vi "G# - SupportMethods.vi"() -> ()   [LabVIEW 2017]
doc: "Support Methods\nThis example demonstrates the use of the G#Object support methods that is always applicable for all G# objects.\n\nBy using the G# Debugger found in Tools->G# Debugger a text log can be followed showing how the objects were created and destroyed."
uses:
  MyDemoClass_class/MyDemoClass.lvclass
  C:/Program Files/National Instruments/LabVIEW 2017/vi.lib/addons/_AddQ/G#Object/G#Object.lvclass
  vi.lib/addons/_AddQ/G#Object/G#Object.lvclass
panel:
  in  "error in (no error)":errorcluster
  out "nr of objects":i32
  out "object name":string
  out "is empty?":bool
  out "string 2":string
  out "string 1":string
  out "is equal 1":bool
  out "is equal 2":bool
  out "class name 2":string
  out "class name 1":string
  out "object ID 2":u32 format="%x"
  out "object ID 1":u32 format="%x"
  out "is instance of":bool
  out "not a refnum? 1":bool
  out "not a refnum? 2":bool
  out "not a refnum? 3":bool
  out "class name 3":string
  out "class path":path
  out "error out":errorcluster
  # "Support Methods\nThis example demonstrates the use of the G#Object support methods that is always applicable for all G# objects.\n\nBy using the G# Debugger found in Tools->G# Debugger a text log can be followed showing how the objects were created and destroyed."
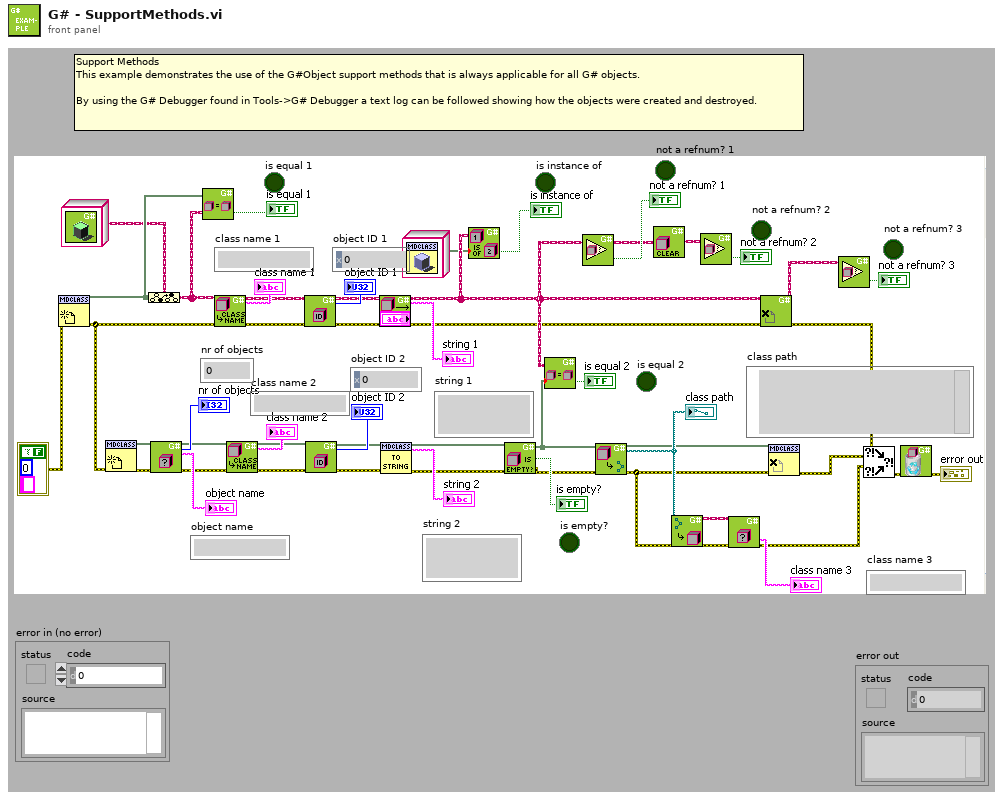
[diagram p1: front panel]
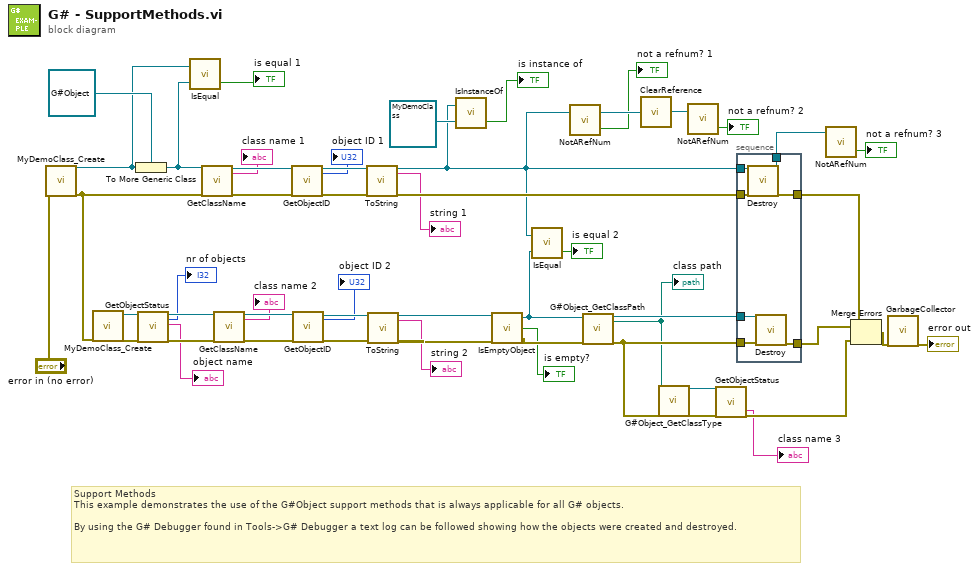
[diagram p0: block diagram]
diagram:
  # "Support Methods\nThis example demonstrates the use of the G#Object support methods that is always applicable for all G# objects.\n\nBy using the G# Debugger found in Tools->G# Debugger a text log can be followed showing how the objects were created and destroyed."
  n1 = call "MyDemoClass_Create.vi"("error in (no error)"="error in (no error)") -> ("reference out"=w12:refnum<class "MyDemoClass.lvclass">, "error out"=w2:errorcluster)  [unwired: 17 in]
  n2 = call "MyDemoClass_Create.vi"("error in (no error)"=w2) -> ("reference out"=w53:refnum<class "MyDemoClass.lvclass">, "error out"=w5:errorcluster)  [unwired: 17 in]
  n3 = To More Generic Class(target class=refnum<class "G#Object.lvclass"> refnum ("reference out"), reference=w12) -> (generic class reference=w11:refnum<class "G#Object.lvclass">)
  n4 = call-dynamic "GetObjectStatus.vi"("reference in"=w53, "error in (no error)"=w5) -> ("# of objects"=→"nr of objects":i32, "reference out"=w52:refnum<class "MyDemoClass.lvclass">, "object name"=→"object name":string, "error out"=w51:errorcluster)  [unwired: 6 in, 8 out]
  n5 = call-dynamic "IsEqual.vi"("is equal to"=w11, "reference in"=w12) -> ("is equal"=→"is equal 1":bool)  [unwired: 1 out]
  n6 = call-dynamic "GetClassName.vi"("reference in"=w11, "error in (no error)"=w2) -> ("reference out"=w18:refnum<class "G#Object.lvclass">, "class name"=→"class name 1":string, "error out"=w19:errorcluster)  [unwired: 13 in, 2 out]
  n7 = call-dynamic "GetClassName.vi"("reference in"=w52, "error in (no error)"=w51) -> ("reference out"=w49:refnum<class "MyDemoClass.lvclass">, "class name"=→"class name 2":string, "error out"=w50:errorcluster)  [unwired: 13 in, 2 out]
  n8 = call-dynamic "GetObjectID.vi"("reference in"=w18, "error in (no error)"=w19) -> ("reference out"=w34:refnum<class "G#Object.lvclass">, "object ID"=→"object ID 1":u32, "error out"=w35:errorcluster)  [unwired: 15 in]
  n9 = call-dynamic "GetObjectID.vi"("reference in"=w49, "error in (no error)"=w50) -> ("reference out"=w40:refnum<class "MyDemoClass.lvclass">, "object ID"=→"object ID 2":u32, "error out"=w48:errorcluster)  [unwired: 15 in]
  n10 = call-dynamic "ToString.vi"("reference in"=w34, "error in (no error)"=w35) -> ("reference out"=w15:refnum<class "G#Object.lvclass">, "string"=→"string 1":string, "error out"=w33:errorcluster)  [unwired: 15 in]
  n11 = call-dynamic "ToString.vi"("reference in"=w40, "error in (no error)"=w48) -> ("reference out"=w37:refnum<class "MyDemoClass.lvclass">, "string"=→"string 2":string, "error out"=w45:errorcluster)  [unwired: 15 in]
  n12 = call-dynamic "IsInstanceOf.vi"("is object instance of"=refnum<class "MyDemoClass.lvclass"> refnum ("reference in"), "reference in"=w15) -> ("is instance of"=→"is instance of":bool)  [unwired: 1 out]
  n13 = call-dynamic "IsEmptyObject.vi"("error in (no error)"=w45, "reference in"=w37) -> ("error out"=w44:errorcluster, "is empty?"=→"is empty?":bool, "reference out"=w14:refnum<class "MyDemoClass.lvclass">)  [unwired: 1 in]
  n14 = call-dynamic "IsEqual.vi"("is equal to"=w14, "reference in"=w15) -> ("is equal"=→"is equal 2":bool)  [unwired: 1 out]
  n15 = call-dynamic "NotARefNum.vi"("reference in"=w15) -> ("not a refnum?"=→"not a refnum? 1":bool, "reference out"=w47:refnum<class "G#Object.lvclass">)  [unwired: 1 in]
  n16 = call-dynamic "G#Object_GetClassPath.vi"("reference in"=w14, "error in (no error)"=w44) -> ("reference out"=w36:refnum<class "MyDemoClass.lvclass">, "class path"=w30:path, "error out"=w31:errorcluster)  [unwired: 15 in]
  "class path" <- w30
  n17 = call-dynamic "ClearReference.vi"("reference in"=w47) -> ("reference out"=w46:refnum<class "G#Object.lvclass">)
  n18 = call "G#Object_GetClassType.vi"("class path"=w30, "error in (no error)"=w31) -> ("reference out"=w27:refnum<class "G#Object.lvclass">, "error out"=w29:errorcluster)  [unwired: 16 in]
  n19 = call-dynamic "NotARefNum.vi"("reference in"=w46) -> ("not a refnum?"=→"not a refnum? 2":bool)  [unwired: 1 in, 1 out]
  n20 = call-dynamic "GetObjectStatus.vi"("reference in"=w27, "error in (no error)"=w29) -> ("class name"=→"class name 3":string, "error out"=w28:errorcluster)  [unwired: 6 in, 10 out]
  n21 = stacked-sequence {
    tunnel: [w60] -> w41
    tunnel: [w59] -> w38
    tunnel: w36 -> [w58]
    tunnel: w33 -> [w57]
    tunnel: w31 -> [w56]
    tunnel: w15 -> [w55]
    tunnel: [w54] -> w6
    frame #0 {
      n22 = call-dynamic "Destroy.vi"("reference in"=w55, "error in (no error)"=w57) -> ("reference out"=w54:refnum<class "G#Object.lvclass">, "error out"=w59:errorcluster)  [unwired: 16 in]
      n23 = call-dynamic "Destroy.vi"("reference in"=w58, "error in (no error)"=w56) -> ("error out"=w60:errorcluster)  [unwired: 16 in, 1 out]
    }
  }
  n24 = call-dynamic "NotARefNum.vi"("reference in"=w6) -> ("not a refnum?"=→"not a refnum? 3":bool)  [unwired: 1 in, 1 out]
  n25 = Merge Errors(w38, w41, w28) -> (w42:errorcluster)
  n26 = call "GarbageCollector.vi"("error in (no error)"=w42) -> ("error out"=→"error out":errorcluster)  [unwired: 16 in, 2 out]
